vi "CCSA RPJ SLJC PR002 SubVI001.vi"(0 "R":u8=160, 1 "TR":u8=10, 2 "TG":u8=10, 3 "TB":u8=10, 5 "G":u8=160, 9 "B":u8=160, 12 "UR":u8, 13 "UG":u8, 14 "UB":u8) -> (4 "ColorSegmentado":u32(colorbox), 15 "binario":bool)   [LabVIEW 2021]
doc: "Realiza la binarización y segmentación de la imagen, a partir de obtener los valores RGB de una imagen y colocar los umbrales para detección."
panel:
  # "CUEVAS CERÓN SERGIO ALBERTO\nREYES PÉREZ JAVIER\nSALCEDO LICEA JUAN CARLOS"
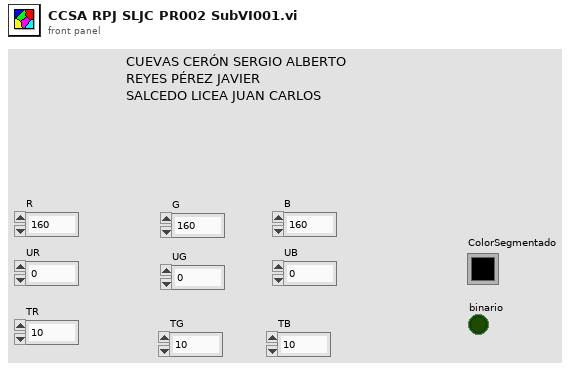
[diagram p1: front panel]
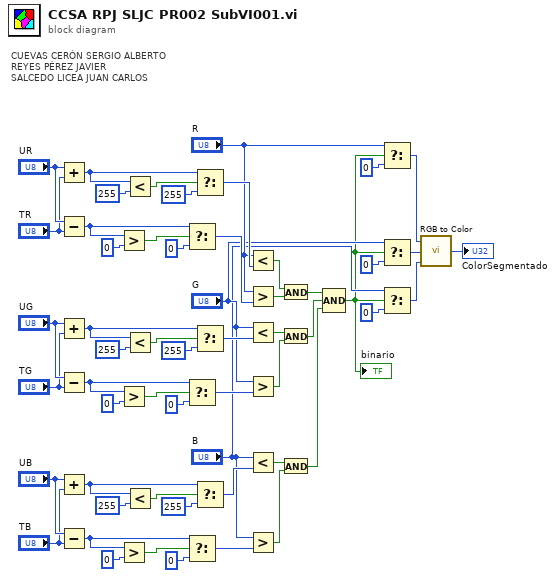
[diagram p0: block diagram]
diagram:
  # "CUEVAS CERÓN SERGIO ALBERTO\nREYES PÉREZ JAVIER\nSALCEDO LICEA JUAN CARLOS"
  n1 = Add(x="UR", y="TR") -> (x+y=w29:u8)
  n2 = Subtract(x="UR", y="TR") -> (x-y=w33:u8)
  n3 = Add(x="UG", y="TG") -> (x+y=w42:u8)
  n4 = Subtract(x="UG", y="TG") -> (x-y=w46:u8)
  n5 = Add(x="UB", y="TB") -> (x+y=w16:u8)
  n6 = Subtract(x="UB", y="TB") -> (x-y=w20:u8)
  n7 = Greater?(x=w33, y=u8 0) -> (0:w35:bool)
  n8 = Greater?(x=w46, y=u8 0) -> (0:w48:bool)
  n9 = Greater?(x=w20, y=u8 0) -> (0:w22:bool)
  n10 = Less?(x=w29, y=u8 255) -> (x < y?=w30:bool)
  n11 = Less?(x=w42, y=u8 255) -> (x < y?=w43:bool)
  n12 = Less?(x=w16, y=u8 255) -> (x < y?=w17:bool)
  n13 = Select(t=w33, s=w35, f=u8 0) -> (s? t:f=w32:u8)
  n14 = Select(t=w46, s=w48, f=u8 0) -> (s? t:f=w45:u8)
  n15 = Select(t=w20, s=w22, f=u8 0) -> (s? t:f=w19:u8)
  n16 = Select(t=w29, s=w30, f=u8 255) -> (s? t:f=w27:u8)
  n17 = Select(t=w42, s=w43, f=u8 255) -> (s? t:f=w40:u8)
  n18 = Select(t=w16, s=w17, f=u8 255) -> (s? t:f=w14:u8)
  n19 = Less?(x="R", y=w27) -> (x < y?=w39:bool)
  n20 = Greater?(x="R", y=w32) -> (0:w38:bool)
  n21 = Less?(x="G", y=w40) -> (x < y?=w54:bool)
  n22 = Greater?(x="G", y=w45) -> (0:w53:bool)
  n23 = Less?(x="B", y=w14) -> (x < y?=w26:bool)
  n24 = Greater?(x="B", y=w19) -> (0:w25:bool)
  n25 = And(x=w39, y=w38) -> (x .and. y?=w11:bool)
  n26 = And(x=w54, y=w53) -> (x .and. y?=w12:bool)
  n27 = And(x=w26, y=w25) -> (x .and. y?=w13:bool)
  n28 = Compound Arithmetic op=AND(w11, w12, w13) -> (w4:bool)
  "binario" <- w4
  n29 = Select(t="R", s=w4, f=u8 0) -> (s? t:f=w7:u8)
  n30 = Select(t="G", s=w4, f=u8 0) -> (s? t:f=w6:u8)
  n31 = Select(t="B", s=w4, f=u8 0) -> (s? t:f=w5:u8)
  n32 = call <vilib>:"RGB to Color.vi"("B"=w5, "G"=w6, "R"=w7) -> ("Color"=→"ColorSegmentado":u32)
